vi "Update Property.vi"(8 "error in (no error)":errorcluster, 9 "Value":variant, 10 "Name":string, 11 "TimestampPanel in":refnum<class "TimestampPanel.lvclass">) -> (0 "error out":errorcluster, 3 "TimestampPanel out":refnum<class "TimestampPanel.lvclass">)   [LabVIEW 2020, in "Conditum-Tools.lvlib" / "TimestampPanel.lvclass"]
uses:
  TimestampPanel.lvclass
  TimestampPanel.lvclass/TimestampPanel.ctl
  Conditum-Clone/Columns/Timestamp/Timestamp.lvclass
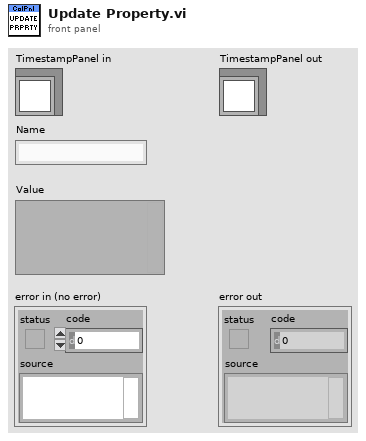
[diagram p1: front panel]
types:
  T1 = typedef "Conditu2.lvlib/Columns.lvlib/Timestamp.lvclass/Definition.ctl" = cluster{"Default":timestamp}
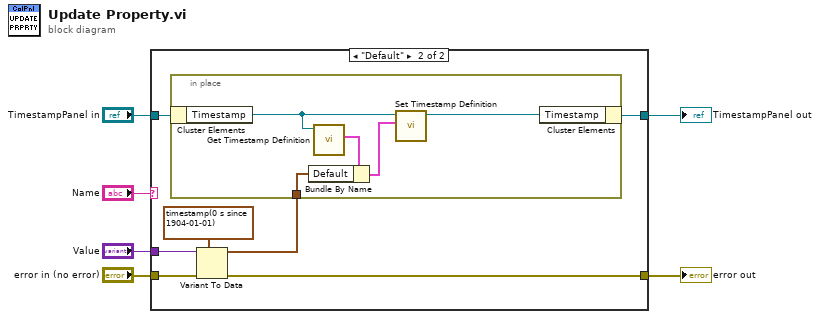
[diagram p0: block diagram]
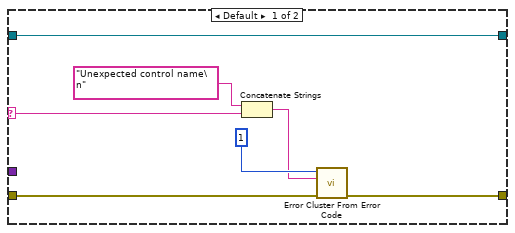
[diagram p2: hidden frame]
diagram:
  n1 = case shown="\"Default\"" "Name" {
    selector: "Name" -> [w9 _]
    tunnel: "Value" -> [_ w20]
    tunnel: "TimestampPanel in" -> [w7 w17]
    tunnel: "error in (no error)" -> [w13 w19]
    tunnel: [w12 w18] -> w4
    tunnel: [w7 w15] -> w5
    frame Default {
      n2 = Concatenate Strings("Unexpected control name\n" ("format string"), w9) -> (w8:string)
      n3 = call <vilib>:"Error Cluster From Error Code.vi"("error in (no error)"=w13, "error message (\"\")"=w8, "error code (0)"=1) -> ("error out"=w12:errorcluster)  [unwired: 6 in]
    }
    frame "Default" {
      n4 = Variant To Data(error in=w19, type=timestamp(0 s since 1904-01-01), Variant=w20) -> (data=w16:timestamp, error out=w18:errorcluster)
      n5 = in-place {
        in-place-border: w16 -> [w24]
        n6 = in-place-cluster #1(w17) -> ("Timestamp"=w23:refnum<class "Timestamp.lvclass">)
        n7 = call "Get Timestamp Definition.vi"("Timestamp in"=w23) -> ("Definition"=w25:T1)  [unwired: 10 in]
        n8 = Bundle By Name(cluster=w25, "Default"=w24) -> (w22:T1)
        n9 = call "Set Timestamp Definition.vi"("Timestamp Definition"=w22, "Timestamp in"=w23) -> ("Timestamp out"=w21:refnum<class "Timestamp.lvclass">)  [unwired: 9 in]
        n10 = in-place-cluster #1("Timestamp"=w21) -> (w15:refnum<class "TimestampPanel.lvclass">)
      }
    }
  }
  "error out" <- w4
  "TimestampPanel out" <- w5
